vi "Periodic Tasks.vi"(8 "error in":errorcluster) -> ()   [LabVIEW 2014]
doc: "This VI runs in parallel to other tasks. It can contain as many user-defined periodic loops as you need. These can carry out PID or other sorts of timed response."
uses:
  <vilib>/Rock Robotics/Network Tables/SD Read Boolean.vi
  Begin/Global Variables.vi
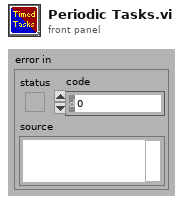
[diagram p1: front panel]
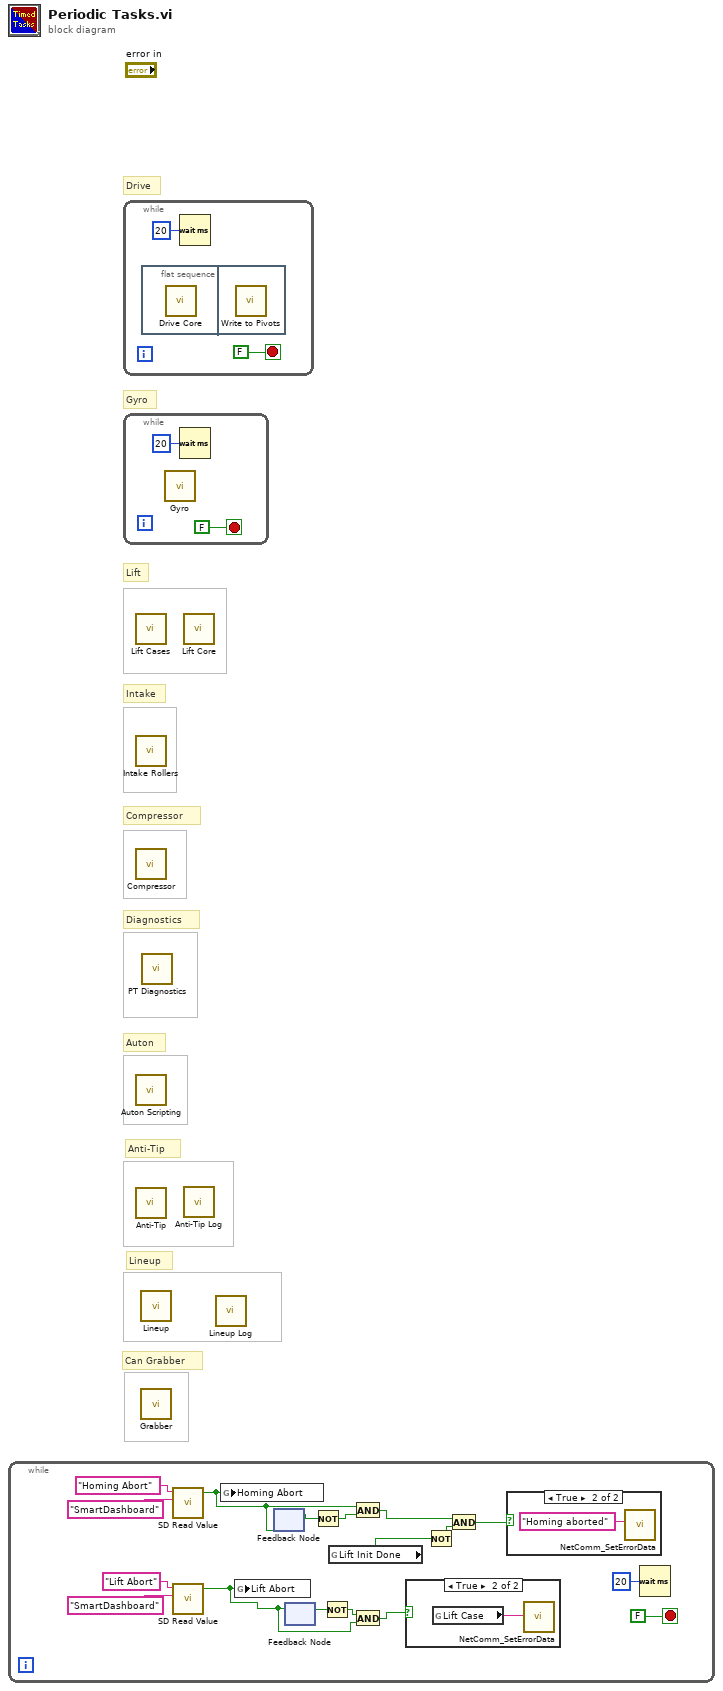
[diagram p0: block diagram]
diagram:
  # "Can Grabber"
  # "Lineup"
  # "Anti-Tip"
  # "Auton"
  # "Drive"
  # "Gyro"
  # "Diagnostics"
  # "Compressor"
  # "Intake"
  # "Lift"
  n1 = while {
    stop <- FALSE stop-if-true
    n2 = call-poly <vilib>:"SD Read Value.vi"("Table Prefix"="SmartDashboard", "Name"="Homing Abort") -> ("Boolean"=w6:bool)  [unwired: 7 in, 2 out]
    n3 = call-poly <vilib>:"SD Read Value.vi"("Table Prefix"="SmartDashboard", "Name"="Lift Abort") -> ("Boolean"=w2:bool)  [unwired: 7 in, 2 out]
    n4 = global write "Global Variables.vi" "Homing Abort"(w6) -> ()
    n5 = global write "Global Variables.vi" "Lift Abort"(w2) -> ()
    n6 = feedback #1() -> (w8:bool)  [unwired: 1 in]
    n7 = feedback-in #1(w6) -> ()
    n8 = feedback #2() -> (w4:bool)  [unwired: 1 in]
    n9 = feedback-in #2(w2) -> ()
    n10 = Not(x=w8) -> (.not. x?=w7:bool)
    n11 = Not(x=w4) -> (.not. x?=w3:bool)
    n12 = global read "Global Variables.vi" "Lift Init Done"() -> (w10:bool)
    n13 = And(x=w6, y=w7) -> (x .and. y?=w5:bool)
    n14 = And(x=w3, y=w2) -> (x .and. y?=w1:bool)
    n15 = case shown="True" w1 {
      frame False {
      }
      frame True {
        n16 = global read "Global Variables.vi" "Lift Case"() -> (w18:string)
        n17 = call <vilib>:"NetComm_SetErrorData.vi"("Error Data"=w18) -> ()  [unwired: 3 in, 8 out]
      }
    }
    n18 = Not(x=w10) -> (.not. x?=w11:bool)
    n19 = And(x=w5, y=w11) -> (x .and. y?=w9:bool)
    n20 = case shown="True" w9 {
      frame False {
      }
      frame True {
        n21 = call <vilib>:"NetComm_SetErrorData.vi"("Error Data"="Homing aborted") -> ()  [unwired: 3 in, 8 out]
      }
    }
    n22 = Wait (ms)(milliseconds to wait=u32 20) -> ()  [unwired: 1 out]
  }
  n23 = while {
    stop <- FALSE stop-if-true
    n24 = flat-sequence {
      frame #0 {
        n25 = call "Drive Core.vi"() -> ()  [unwired: 12 in]
      }
      frame #1 {
        n26 = call "Write to Pivots.vi"() -> ()  [unwired: 12 in]
      }
    }
    n27 = Wait (ms)(milliseconds to wait=u32 20) -> ()  [unwired: 1 out]
  }
  n28 = while {
    stop <- FALSE stop-if-true
    n29 = call "Gyro.vi"() -> ()  [unwired: 12 in]
    n30 = Wait (ms)(milliseconds to wait=u32 20) -> ()  [unwired: 1 out]
  }
  n31 = call "Lift Cases.vi"() -> ()  [unwired: 12 in]
  n32 = call "Intake Rollers.vi"() -> ()  [unwired: 12 in]
  n33 = call "Compressor.vi"() -> ()  [unwired: 12 in]
  n34 = call "Auton Scripting.vi"() -> ()  [unwired: 12 in]
  n35 = call "Anti-Tip.vi"() -> ()  [unwired: 12 in]
  n36 = call "Lineup.vi"() -> ()  [unwired: 12 in]
  n37 = call "Grabber.vi"() -> ()  [unwired: 12 in]
  n38 = call "PT Diagnostics.vi"() -> ()  [unwired: 12 in]
  n39 = call "Lift Core.vi"() -> ()  [unwired: 12 in]
  n40 = call "Anti-Tip Log.vi"() -> ()  [unwired: 12 in]
  n41 = call "Lineup Log.vi"() -> ()  [unwired: 12 in]
